vi "Do Request.vi"(7 "Processing In":refnum<class "Processing.lvclass">, 11 "Registration in":refnum<class "Registration.lvclass">) -> (0 "error out":errorcluster, 5 "Processing":refnum<class "Processing.lvclass">)   [LabVIEW 2020, in "Summer of LabVIEW.lvlib" / "Registration.lvclass"]
uses:
  Registration.lvclass
  <vilib>/IlluminatedG/IG HTTP Server/HTTP Server/Processing/Processing.lvclass
  Data Types/Registration JSON.ctl
  <vilib>/IlluminatedG/IG HTTP Server/HTTP Server/Processing/Processing.lvclass/Processing.ctl
  User DB/User DB.lvclass
  SOL User/SOL User.lvclass
  <vilib>/IlluminatedG/IG HTTP Server/HTTP Server/Password Encoder/Password Encoder.lvclass
  eb8f0320-88f6-4f3e-bd1c-fbb23804af65.vi
  40b538c3-a1ee-4dd7-9a33-91208dd704e8.vi
  eb8f0320-88f6-4f3e-bd1c-fbb23804af65.vi/9528e9df-aefc-4ce0-9221-106a337fd3b6.vi
  40b538c3-a1ee-4dd7-9a33-91208dd704e8.vi/9528e9df-aefc-4ce0-9221-106a337fd3b6.vi
  <vilib>/IlluminatedG/IG HTTP Server/HTTP Server/Values/Get Arg Map.vi
  <vilib>/Utility/error.llb/Error Cluster From Error Code.vi
  Registration.lvclass/Registration.ctl
  <vilib>/IlluminatedG/IG HTTP Utils/HTTP Utils/Request/Request.lvclass
  Summer of LabVIEW.lvlib
  <vilib>/IlluminatedG/IG HTTP Utils/HTTP Utils/Response/Response.lvclass
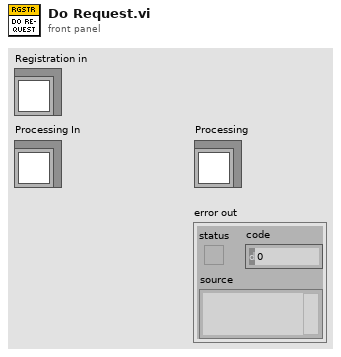
[diagram p1: front panel]
types:
  T1 = typedef "Summer of LabVIEW.lvlib/Registration JSON.ctl" = cluster{"email":string, "password":string, "first_name":string, "last_name":string, "department":string}
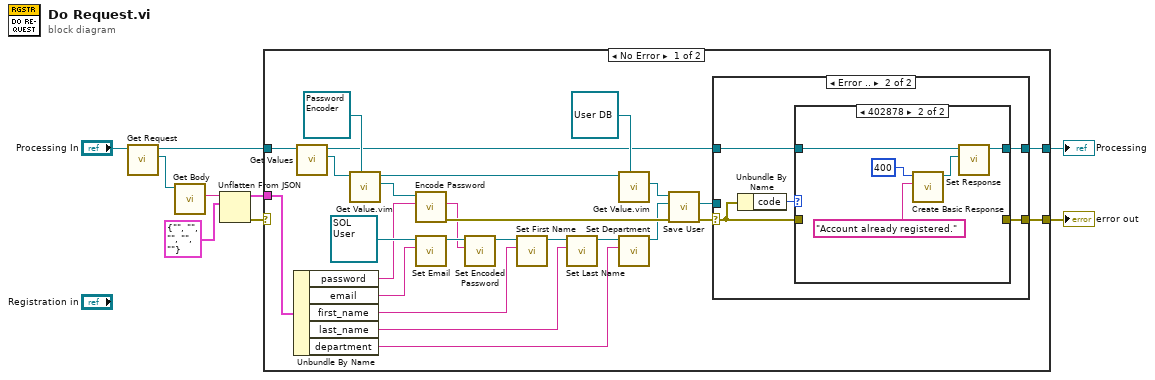
[diagram p0: block diagram]
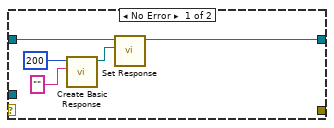
[diagram p2: hidden frame]
diagram:
  n1 = call <vilib>:"Get Request.vi"("Processing in"="Processing In") -> ("Request"=w6:refnum<class "Request.lvclass">, "Processing out"=w7:refnum<class "Processing.lvclass">)  [unwired: 9 in]
  n2 = call <vilib>:"Get Body.vi"("Request in"=w6) -> ("Body"=w5:string)  [unwired: 8 in, 2 out]
  n3 = Unflatten From JSON(JSON string=w5, type and defaults=T1 {"email"="", "password"="", "first_name"="", "last_name"="", "department"=""} ("Registration JSON")) -> (value=w2:T1, error out=w3:errorcluster)  [unwired: 5 in]
  n4 = case shown="No Error" w3 {
    selector: w3 -> [_ w54]
    tunnel: [w11 w53] -> w9
    tunnel: w7 -> [w33 w53]
    tunnel: w2 -> [w32 _]
    tunnel: [w10 w54] -> w1
    frame No Error {
      n5 = Unbundle By Name(w32) -> ("password"=w26:string, "email"=w30:string, "first_name"=w22:string, "last_name"=w20:string, "department"=w18:string)
      n6 = call <vilib>:"Get Values.vi"("Processing in"=w33) -> ("Values"=w29:refnum<class "Values.lvclass">, "Processing out"=w12:refnum<class "Processing.lvclass">)  [unwired: 9 in]
      n7 = call "Get Value.vim"("Type / Server / Service (String)"=refnum<class "Password Encoder.lvclass"> refnum ("HTTP Server.lvlib:Password Encoder.lvclass"), "Arguments in"=w29) -> ("Value"=w27:refnum<class "Password Encoder.lvclass">, "Arguments out"=w17:refnum<class "Values.lvclass">)  [unwired: 7 in, 1 out]
      n8 = call-dynamic "Encode Password.vi"("Plain Password"=w26, "Password Encoder in"=w27) -> ("error out"=w35:errorcluster, "Encoded Password"=w24:string)  [unwired: 7 in, 1 out]
      n9 = call "Set Email.vi"("Email"=w30, "SOL User in"=refnum<class "SOL User.lvclass"> refnum) -> ("SOL User out"=w25:refnum<class "SOL User.lvclass">)  [unwired: 8 in, 1 out]
      n10 = call "Set Encoded Password.vi"("Encoded Password"=w24, "SOL User in"=w25) -> ("SOL User out"=w23:refnum<class "SOL User.lvclass">)  [unwired: 8 in, 1 out]
      n11 = call "Set First Name.vi"("First Name"=w22, "SOL User in"=w23) -> ("SOL User out"=w21:refnum<class "SOL User.lvclass">)  [unwired: 8 in, 1 out]
      n12 = call "Set Last Name.vi"("Last Name"=w20, "SOL User in"=w21) -> ("SOL User out"=w19:refnum<class "SOL User.lvclass">)  [unwired: 8 in, 1 out]
      n13 = call "Get Value.vim"("Type / Server / Service (String)"=refnum<class "User DB.lvclass"> refnum ("SOL:User DB.lvclass"), "Arguments in"=w17) -> ("Value"=w16:refnum<class "User DB.lvclass">)  [unwired: 7 in, 2 out]
      n14 = call "Set Department.vi"("Department"=w18, "SOL User in"=w19) -> ("SOL User out"=w15:refnum<class "SOL User.lvclass">)  [unwired: 8 in, 1 out]
      n15 = call "Save User.vi"("error in (no error)"=w35, "User In"=w15, "User DB in"=w16) -> ("error out"=w14:errorcluster, "User"=w13:refnum<class "SOL User.lvclass">)  [unwired: 6 in, 1 out]
      n16 = case shown="Error .." w14 {
        selector: w14 -> [_ w42]
        tunnel: w13 -> [_ _]
        tunnel: w12 -> [w36 w44]
        tunnel: [w40 w43] -> w11
        tunnel: [_ w41] -> w10
        frame No Error {
          n17 = call <vilib>:"Create Basic Response.vi"("Payload"="", "Status Code"=u16 200) -> ("Response out"=w37:refnum<class "Response.lvclass">)  [unwired: 8 in, 1 out]
          n18 = call <vilib>:"Set Response.vi"("Response"=w37, "Processing in"=w36) -> ("Processing out"=w40:refnum<class "Processing.lvclass">)  [unwired: 9 in]
        }
        frame Error {
          n19 = Unbundle By Name(w42) -> ("code"=w45:i32)
          n20 = case shown="402878" w45 {
            tunnel: w44 -> [w47 w52]
            tunnel: [w47 w51] -> w43
            tunnel: w42 -> [w46 _]
            tunnel: [w46 _] -> w41
            frame Default {
            }
            frame 402878 {
              n21 = call <vilib>:"Create Basic Response.vi"("Payload"="Account already registered.", "Status Code"=u16 400) -> ("Response out"=w50:refnum<class "Response.lvclass">)  [unwired: 8 in, 1 out]
              n22 = call <vilib>:"Set Response.vi"("Response"=w50, "Processing in"=w52) -> ("Processing out"=w51:refnum<class "Processing.lvclass">)  [unwired: 9 in]
            }
          }
        }
      }
    }
    frame Error {
    }
  }
  "error out" <- w1
  "Processing" <- w9
